vi "TabControl.vi"() -> ()   [LabVIEW 2021]
panel:
  in  "stop":bool
  in  "Tab Control":enum32{"Page 1", "Page 2"}(tab)
  out "Multi":dbl
  out "Add":dbl
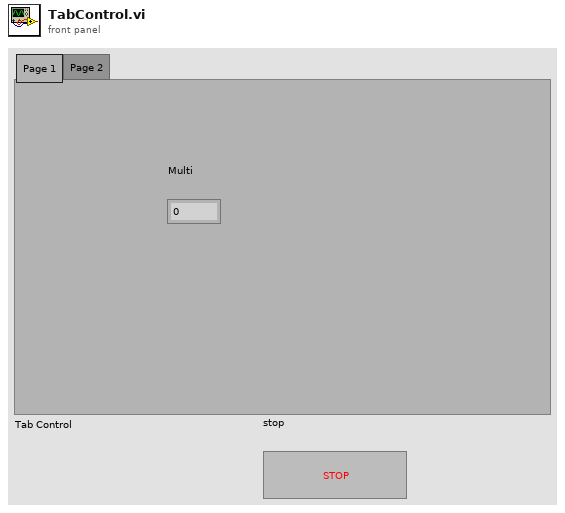
[diagram p1: front panel]
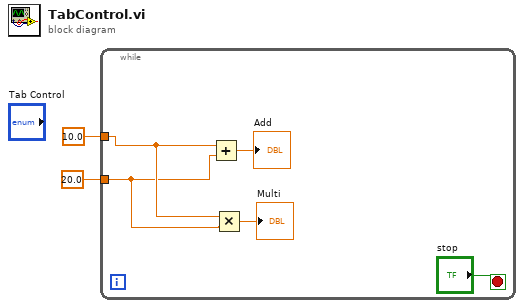
[diagram p0: block diagram]
diagram:
  n1 = while {
    tunnel: 10.0 -> [w5]
    tunnel: 20.0 -> [w4]
    stop <- "stop" stop-if-true
    n2 = Add(x=w5, y=w4) -> (x+y=→"Add":dbl)
    n3 = Multiply(x=w5, y=w4) -> (x*y=→"Multi":dbl)
  }
